vi "Distance to Hub.vi"() -> (1 "Sees Tag?":bool, 3 "Distance to Hub (ft)":dbl)   [LabVIEW 2025]
uses:
  <vilib>/Rock Robotics/Network Tables/NT Read Float Array.vi
  <vilib>/Rock Robotics/Network Tables/NT Read Number.vi
panel:
  in  "Offset (ft)":dbl
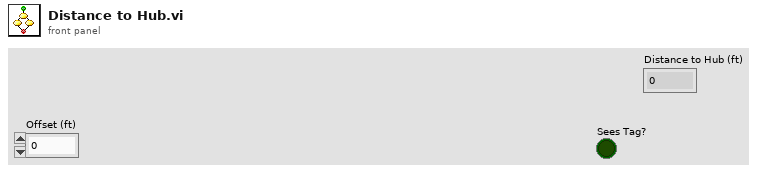
[diagram p1: front panel]
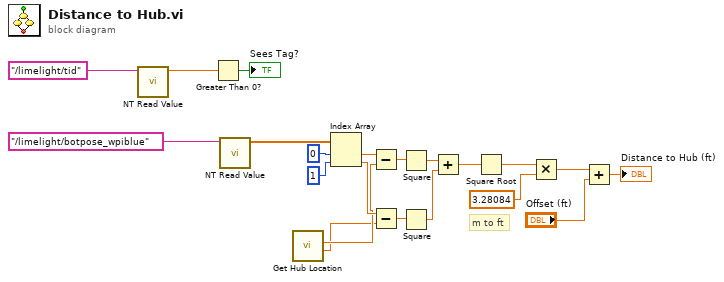
[diagram p0: block diagram]
diagram:
  # "m to ft"
  n1 = call-poly <vilib>:"NT Read Value.vi"("name"="/limelight/tid") -> ("value"=w5:dbl)  [unwired: 8 in, 2 out]
  n2 = Greater Than 0?(x=w5) -> (x > 0?=→"Sees Tag?":bool)
  n3 = call-poly <vilib>:"NT Read Value.vi"("name"="/limelight/botpose_wpiblue") -> ("value"=w20:sgl[])  [unwired: 8 in, 2 out]
  n4 = call "Get Hub Location.vi"() -> ("Hub Y"=w1:dbl, "Hub X"=w2:dbl)  [unwired: 10 in]
  n5 = Index Array(array=w20, index #1=0 ("index"), index #2=1 ("index")) -> (element #1=w17:sgl, element #2=w15:sgl)
  n6 = Subtract(x=w17, y=w2) -> (x-y=w16:dbl)
  n7 = Subtract(x=w15, y=w1) -> (x-y=w14:dbl)
  n8 = Square(x=w16) -> (x^2=w12:dbl)
  n9 = Square(x=w14) -> (x^2=w11:dbl)
  n10 = Add(x=w12, y=w11) -> (x+y=w13:dbl)
  n11 = Square Root(x=w13) -> (sqrt(x)=w9:dbl)
  n12 = Multiply(x=w9, y=3.28084) -> (x*y=w8:dbl)
  n13 = Add(x=w8, y="Offset (ft)") -> (x+y=→"Distance to Hub (ft)":dbl)
